vi "Scale Window.vi"(0 "VI in":refnum<vi>, 11 "error in (no error)":errorcluster) -> (4 "VI out":refnum<vi>, 15 "error out":errorcluster)   [LabVIEW 2016, in "LV Doc.lvclass"]
uses:
  LV Doc.lvclass
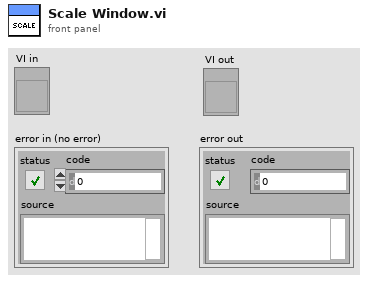
[diagram p1: front panel]
types:
  T1 = enum16{"No Scaling", "Scale All Objects", "Scale Single Object"}
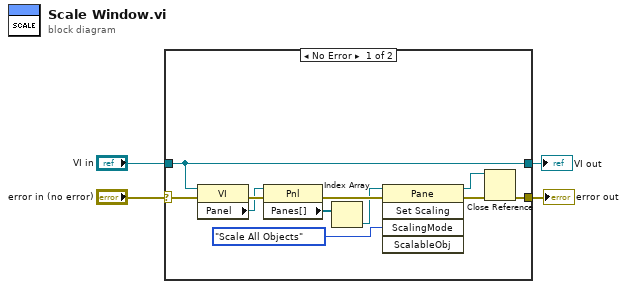
[diagram p0: block diagram]
diagram:
  n1 = case shown="No Error" "error in (no error)" {
    selector: "error in (no error)" -> [w14 w17]
    tunnel: [w7 w17] -> w4
    tunnel: "VI in" -> [w5 w16]
    tunnel: [w5 w16] -> w1
    frame No Error {
      n2 = property class="VI"(reference=w5, error in=w14) -> (error out=w12:errorcluster, "Panel"=w8:refnum<vi>)  [unwired: 1 out]
      n3 = property class="Pnl"(reference=w8, error in=w12) -> (error out=w13:errorcluster, "Panes[]"=w9:refnum<vi>[])  [unwired: 1 out]
      n4 = Index Array(array=w9) -> (element=w10:refnum<vi>)  [unwired: 1 in]
      n5 = invoke class="Pane" method="Set Scaling"(reference=w10, error in=w13, "ScalingMode"=T1."Scale All Objects" ("Scaling Mode")) -> (reference out=w6:refnum<vi>, error out=w15:errorcluster)  [unwired: 2 in, 3 out]
      n6 = Close Reference(reference=w6, error in (no error)=w15) -> (error out=w7:errorcluster)
    }
    frame Error {
    }
  }
  "error out" <- w4
  "VI out" <- w1
